vi "Convert Array from IMPARAMS.vi"(2 "IMPARAMS":T1) -> (16 "Array":u32[](array[numeric]))   [LabVIEW 2013, in "VRI.lvlib"]
uses:
  VRI.lvlib
  _Type Defs/PHCon IMPARAMS.ctl
  _Type Defs/PhInt WBGAIN.ctl
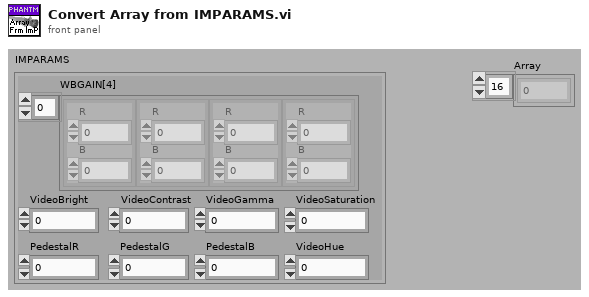
[diagram p1: front panel]
types:
  T1 = typedef "VRI.lvlib/PHCon IMPARAMS.ctl" = cluster{"WBGAIN[4]":T2[], "VideoBright":i32, "VideoContrast":i32, "VideoGamma":sgl, "VideoSaturation":i32, "PedestalR":i32, "PedestalG":i32, "PedestalB":i32, "VideoHue":i32}
  T2 = typedef "VRI.lvlib/PhInt WBGAIN.ctl" = cluster{"R":sgl, "B":sgl}
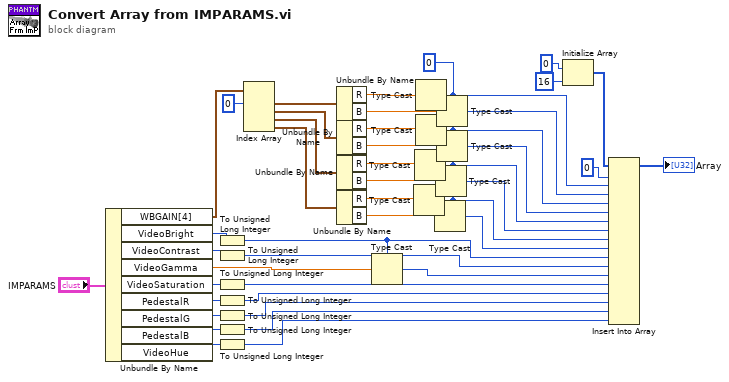
[diagram p0: block diagram]
diagram:
  w3 = u32 0 ("index")
  n1 = Unbundle By Name("IMPARAMS") -> ("WBGAIN[4]"=w44:T2[], "VideoBright"=w34:i32, "VideoContrast"=w33:i32, "VideoGamma"=w5:sgl, "VideoSaturation"=w32:i32, "PedestalR"=w31:i32, "PedestalG"=w30:i32, "PedestalB"=w29:i32, "VideoHue"=w28:i32)
  n2 = To Unsigned Long Integer(number=w34) -> (unsigned 32bit integer=w1:u32)
  n3 = To Unsigned Long Integer(number=w33) -> (unsigned 32bit integer=w2:u32)
  n4 = To Unsigned Long Integer(number=w32) -> (unsigned 32bit integer=w27:u32)
  n5 = To Unsigned Long Integer(number=w31) -> (unsigned 32bit integer=w26:u32)
  n6 = To Unsigned Long Integer(number=w30) -> (unsigned 32bit integer=w25:u32)
  n7 = To Unsigned Long Integer(number=w29) -> (unsigned 32bit integer=w24:u32)
  n8 = To Unsigned Long Integer(number=w28) -> (unsigned 32bit integer=w23:u32)
  n9 = Index Array(array=w44, index #1=0 ("index")) -> (element #1=w42:T2, element #2=w41:T2, element #3=w40:T2, element #4=w39:T2)  [unwired: 3 in]
  n10 = Unbundle By Name(w42) -> ("R"=w21:sgl, "B"=w19:sgl)
  n11 = Unbundle By Name(w41) -> ("R"=w18:sgl, "B"=w17:sgl)
  n12 = Unbundle By Name(w40) -> ("R"=w16:sgl, "B"=w15:sgl)
  n13 = Unbundle By Name(w39) -> ("R"=w14:sgl, "B"=w13:sgl)
  n14 = Type Cast(type=w1, x=w5) -> (*(type *) &x=w4:u32)
  n15 = Type Cast(type=w3, x=w14) -> (*(type *) &x=w7:u32)
  n16 = Type Cast(type=w3, x=w16) -> (*(type *) &x=w9:u32)
  n17 = Type Cast(type=w3, x=w21) -> (*(type *) &x=w20:u32)
  n18 = Type Cast(type=w3, x=w18) -> (*(type *) &x=w11:u32)
  n19 = Type Cast(type=w3, x=w13) -> (*(type *) &x=w6:u32)
  n20 = Type Cast(type=w3, x=w15) -> (*(type *) &x=w8:u32)
  n21 = Type Cast(type=w3, x=w19) -> (*(type *) &x=w12:u32)
  n22 = Type Cast(type=w3, x=w17) -> (*(type *) &x=w10:u32)
  n23 = Initialize Array(u32 0 ("element"), 16 ("dimension size")) -> (w36:u32[])
  n24 = Insert Into Array(array=w36, index=0, new element #1=w20, new element #2=w12, new element #3=w11, new element #4=w10, new element #5=w9, new element #6=w8, new element #7=w7, new element #8=w6, new element #9=w1, new element #10=w2, new element #11=w4, new element #12=w27, new element #13=w26, new element #14=w25, new element #15=w24, new element #16=w23) -> (→"Array":u32[])
